vi "Exit Windows.vi"(9 "show prompt? (T)":bool=TRUE, 10 "force? (F)":bool, 11 "exit function\n(0 - Logoff)":T1(ring)) -> (0 "error out":errorcluster)   [LabVIEW 2011]
doc: "This VI allows you to exit windows in various ways.\n\nexit windows function\n 0 : Logoff\n 1 : Shutdown System\n 2 : Reboot System\n 3 : Force Logoff\n 4 : Power off the system (not supported in all systems)"
panel:
  in  "error in (no error)":errorcluster
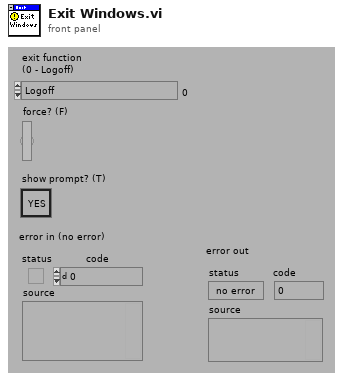
[diagram p1: front panel]
types:
  T1 = enum16{"Logoff", "Shutdown System", "Reboot System", "Poweroff System"}
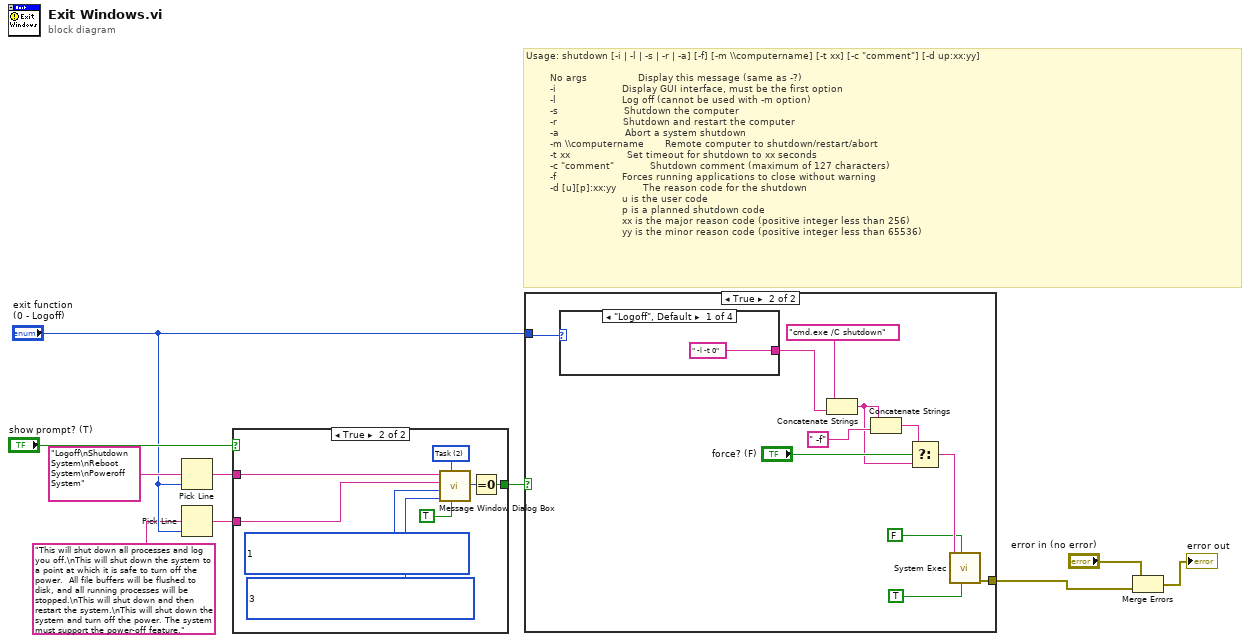
[diagram p0: block diagram]
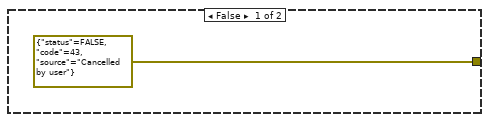
[diagram p2: hidden frame]
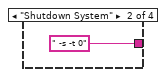
[diagram p3: hidden frame]
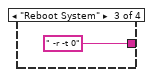
[diagram p4: hidden frame]
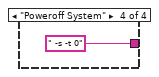
[diagram p5: hidden frame]
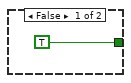
[diagram p6: hidden frame]
diagram:
  # "Usage: shutdown [-i | -l | -s | -r | -a] [-f] [-m \\\\computername] [-t xx] [-c \"comment\"] [-d up:xx:yy]\n\n        No args                 Display this message (same as -?)\n        -i                      Display GUI interface, must be the first option\n        -l                      Log off (cannot be used with -m option)\n        -s                      Shutdown the computer\n        -r                      Shutdown and restart the computer\n        -a                      Abort a system shutdown\n        -m \\\\computername       Remote computer to shutdown/restart/abort\n        -t xx                   Set timeout for shutdown to xx seconds\n        -c \"comment\"            Shutdown comment (maximum of 127 characters)\n        -f                      Forces running applications to close without warning\n        -d [u][p]:xx:yy         The reason code for the shutdown\n                                u is the user code\n                                p is a planned shutdown code\n                                xx is the major reason code (positive integer less than 256)\n                                yy is the minor reason code (positive integer less than 65536)"
  n1 = Pick Line(multi-line string="Logoff\nShutdown System\nReboot System\nPoweroff System", line index="exit function\n(0 - Logoff)") -> (output string=w7:string)  [unwired: 1 out]
  n2 = Pick Line(multi-line string="This will shut down all processes and log you off.\nThis will shut down the system to a point at which it is safe to turn off the power.  All file buffers will be flushed to disk, and all running processes will be stopped.\nThis will shut down and then restart the system.\nThis will shut down the system and turn off the power. The system must support the power-off feature.", line index="exit function\n(0 - Logoff)") -> (output string=w6:string)  [unwired: 1 out]
  n3 = case shown="True" "show prompt? (T)" {
    tunnel: [TRUE w19] -> w9
    tunnel: w7 -> [_ w16]
    tunnel: w6 -> [_ w15]
    frame False {
    }
    frame True {
      w12 = 2 items=["Application", "System", "Task"] ("modality (0)")
      n4 = call "Message Window Dialog Box.vi"("sound? (F)"=TRUE, "modality (0)"=w12, "icon (0:None)"=3, "buttons (0:OK)"=1, "message (\"\")"=w15, "window title (\"\")"=w16) -> ("button pressed"=w18:i32)  [unwired: 1 in, 3 out]
      n5 = Equal To 0?(x=w18) -> (x = 0?=w19:bool)
    }
  }
  n6 = case shown="True" w9 {
    tunnel: "exit function\n(0 - Logoff)" -> [_ w29]
    tunnel: [errorcluster {"status"=FALSE, "code"=43, "source"="Cancelled by user"} ("error out") w31] -> w3
    frame False {
    }
    frame True {
      n7 = case shown="\"Logoff\", Default" w29 {
        tunnel: [" -l -t 0" ("command line") " -s -t 0" ("command line") " -r -t 0" ("command line") " -s -t 0" ("command line")] -> w25
        frame "Logoff", Default {
        }
        frame "Shutdown System" {
        }
        frame "Reboot System" {
        }
        frame "Poweroff System" {
        }
      }
      n8 = Concatenate Strings("cmd.exe /C shutdown" ("command line"), w25) -> (w22:string)
      n9 = Concatenate Strings(w22, " -f" ("command line")) -> (w23:string)
      n10 = Select(t=w23, s="force? (F)", f=w22) -> (s? t:f=w27:string)
      n11 = call <vilib>:"System Exec.vi"("run minimized? (F)"=TRUE, "wait until completion? (T)"=FALSE, "command line"=w27) -> ("error out"=w31:errorcluster)  [unwired: 3 in, 5 out]
    }
  }
  n12 = Merge Errors("error in (no error)", w3) -> (→"error out":errorcluster)
